vi "Login usuario.vi"() -> (1 "categoria out":string, 2 "Usuario y Pass OK?":bool, 3 "Usuario out":string)   [LabVIEW 2018]
uses:
  <vilib>/RAFA Solutions/Harmony UI Controls Kit/String & Path/String Control.ctl
  <vilib>/RAFA Solutions/Harmony UI Controls Kit/Boolean/OK Button.ctl
  <vilib>/RAFA Solutions/Harmony UI Controls Kit/Boolean/Cancel Button.ctl
  <vilib>/RAFA Solutions/Harmony UI Controls Kit/Flat UI Design.lvlib
panel:
  out "build":string
  in  "Cancel":T1
  in  "OK":T2
  in  "Contraseña":T3
  in  "Usuario":T3
  # "BIENVENIDO"
  # "Sistema de Monitoreo de Calidad de Energía"
  # "www.dts.cl"
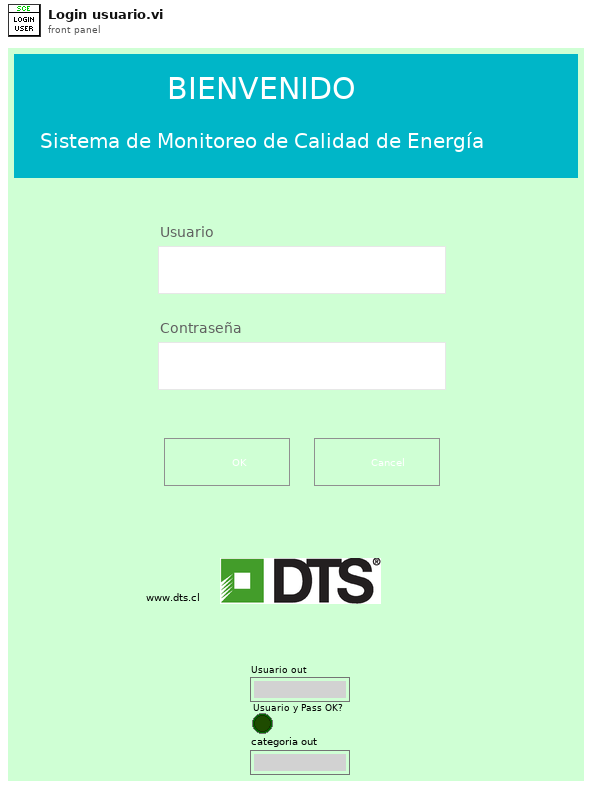
[diagram p1: front panel]
types:
  T1 = typedef "Flat UI Design.lvlib/Cancel Button.ctl" = bool
  T2 = typedef "Flat UI Design.lvlib/OK Button.ctl" = bool
  T3 = typedef "Flat UI Design.lvlib/String Control.ctl" = string
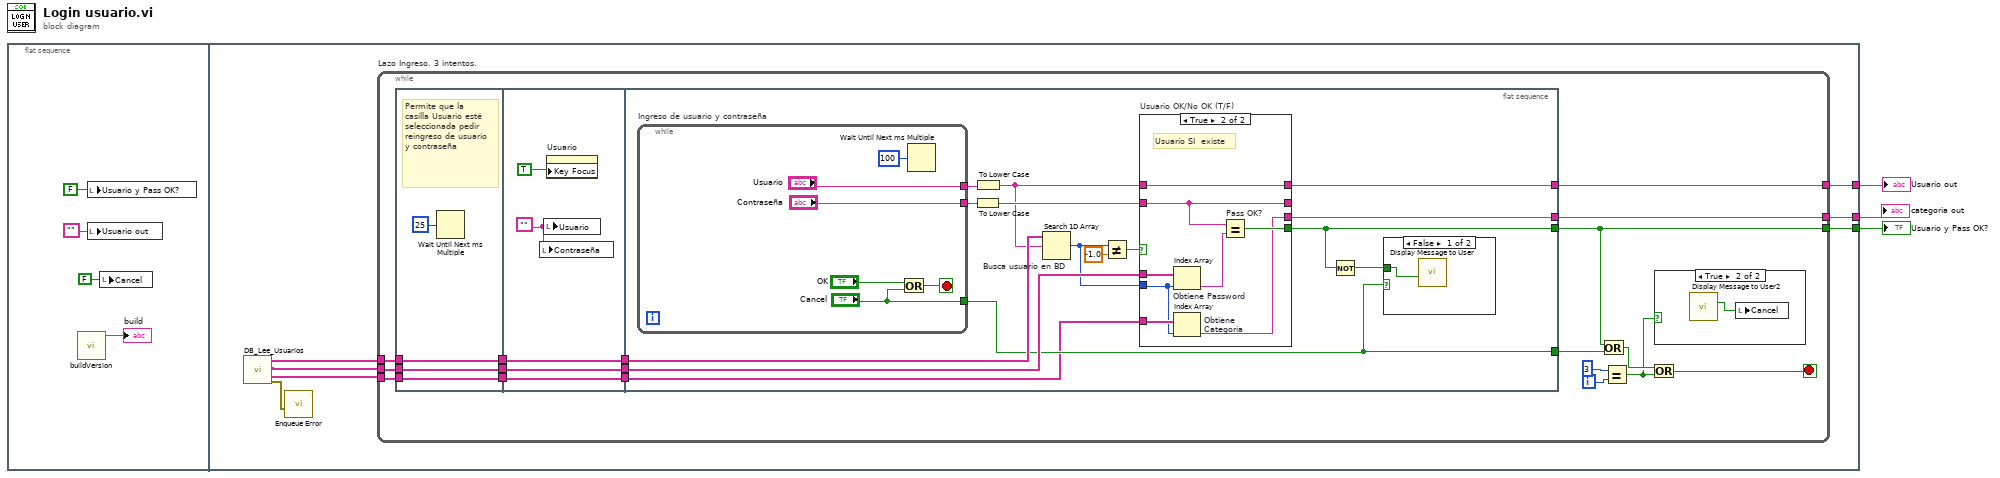
[diagram p0: block diagram]
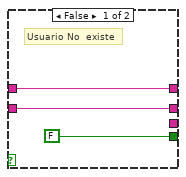
[diagram p4: hidden frame]
diagram:
  n1 = flat-sequence {
    tunnel: [w14] -> w2
    tunnel: [w13] -> w3
    tunnel: [w12] -> w1
    frame #0 {
      n2 = call "buildVersion.vi"() -> ("build"=→"build":string)  [unwired: 11 in]
      n3 = local write "Usuario y Pass OK?"(FALSE ("Usuario y Pass OK?")) -> ()
      n4 = local write "Usuario out"("") -> ()
      n5 = local write "Cancel"(T1 FALSE ("Cancel")) -> ()
    }
    frame #1 {
      n6 = call "DB_Lee_Usuarios.vi"() -> ("error out"=w8:errorcluster, "categorias"=w9:string[], "pass"=w10:string[], "usuarios"=w11:string[])  [unwired: 8 in]
      n7 = call "Enqueue Error.vi"("error in"=w8) -> ()  [unwired: 9 in, 2 out]
      n8 = while "Lazo Ingreso. 3 intentos." {
        tunnel: w11 -> [w29]
        tunnel: w10 -> [w28]
        tunnel: w9 -> [w17]
        tunnel: [w27] -> w14
        tunnel: [w24] -> w13
        tunnel: [w16] -> w12
        i -> [w32]
        stop <- w30 stop-if-true
        n9 = flat-sequence {
          tunnel: w28 -> [w36]
          tunnel: w29 -> [w37]
          tunnel: [w37] -> w21
          tunnel: [w36] -> w20
          tunnel: [w34] -> w18
          tunnel: w17 -> [w34]
          tunnel: [w42] -> w23
          tunnel: [w41] -> w22
          tunnel: w21 -> [w42]
          tunnel: w20 -> [w41]
          tunnel: [w38] -> w19
          tunnel: w18 -> [w38]
          tunnel: [w48] -> w27
          tunnel: [w45] -> w25
          tunnel: [w46] -> w24
          tunnel: w23 -> [w55]
          tunnel: w22 -> [w54]
          tunnel: w19 -> [w44]
          tunnel: [w43] -> w16
          frame #0 {
            # "Permite que la casilla Usuario esté seleccionada pedir reingreso de usuario y contraseña"
            n10 = Wait Until Next ms Multiple(millisecond multiple=u32 25) -> ()  [unwired: 1 out]
          }
          frame #1 {
            w40 = ""
            n11 = local write "Contraseña"(w40) -> ()
            n12 = local write "Usuario"(w40) -> ()
            n13 = property on="Usuario" class="Str (strict)"("Key Focus"=TRUE) -> ()  [unwired: 2 in, 2 out]
          }
          frame #2 {
            n14 = while "Ingreso de usuario y contraseña" {
              tunnel: ["Usuario"] -> w57
              tunnel: ["Contraseña"] -> w56
              tunnel: ["Cancel"] -> w45
              stop <- w74 stop-if-true
              n15 = Or(x="OK", y="Cancel") -> (x .or. y?=w74:T2)
              n16 = Wait Until Next ms Multiple(millisecond multiple=u32 100) -> ()  [unwired: 1 out]
            }
            n17 = To Lower Case(string=w56) -> (all lower case string=w51:T3)
            n18 = To Lower Case(string=w57) -> (all lower case string=w49:T3)
            n19 = Search 1D Array "Busca usuario en BD"(1D array=w55, element=w49) -> (index of element=w50:i32)  [unwired: 1 out]
            n20 = Not Equal?(x=w50, y=-1.0) -> (x != y?=w52:bool)
            n21 = case "Usuario OK/No OK (T/F)" shown="True" w52 {
              tunnel: w54 -> [_ w69]
              tunnel: w51 -> [w60 w62]
              tunnel: [FALSE w67] -> w46
              tunnel: w50 -> [_ w64]
              tunnel: [w60 w62] -> _
              tunnel: [w59 w66] -> w48
              tunnel: w49 -> [w59 w66]
              tunnel: w44 -> [_ w65]
              tunnel: [_ w63] -> w43
              frame False {
                # "Usuario No  existe"
              }
              frame True {
                # "Usuario SI  existe"
                n22 = Index Array "Obtiene Password"(array=w69, index=w64) -> (element=w68:string)
                n23 = Index Array "Obtiene\nCategoría"(array=w65, index=w64) -> (element=w63:string)
                n24 = Equal? "Pass OK?"(x=w62, y=w68) -> (x = y?=w67:bool)
              }
            }
            n25 = Not(x=w46) -> (.not. x?=w47:bool)
            n26 = case shown="False" w45 {
              tunnel: w47 -> [w58 _]
              frame False {
                n27 = call "Display Message to User"("Enable"=w58) -> ()  [unwired: 2 in, 9 out]
              }
              frame True {
              }
            }
          }
        }
        n28 = Or(x=w24, y=w25) -> (x .or. y?=w26:T1)
        n29 = Equal?(x=3, y=w32) -> (x = y?=w15:bool)
        n30 = Or(x=w26, y=w15) -> (x .or. y?=w30:T1)
        n31 = case shown="True" w15 {
          frame False {
          }
          frame True {
            n32 = call "Display Message to User2"() -> ("OK"=w33:bool)  [unwired: 3 in, 8 out]
            n33 = local write "Cancel"(w33) -> ()
          }
        }
      }
    }
  }
  "Usuario out" <- w2
  "Usuario y Pass OK?" <- w3
  "categoria out" <- w1
